vi "Launch Process.vi"(8 "error in (no error)":errorcluster, 10 "TopLevel":refnum<class "TopLevel.lvclass">, 11 "Database in":refnum<class "Database.lvclass">) -> (0 "error out":errorcluster, 1 "timed out?":bool, 2 "sync from process?":bool, 3 "Database out":refnum<class "Database.lvclass">)   [LabVIEW 2022 SP3, in "Database.lvclass"]
doc: "Developed by Kevin Thompson\nkevin@thompsonengineering.net\n\nCopyright 2018\nThompson Engineering, LLC"
uses:
  Database.lvclass
  TopLevel/TopLevel.lvclass
  Process.vi
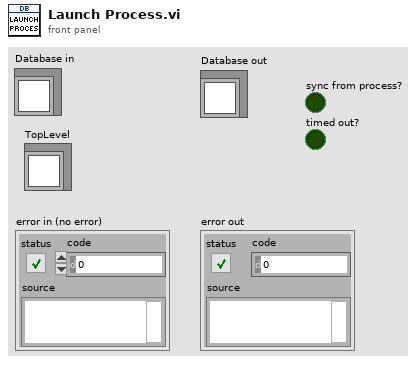
[diagram p1: front panel]
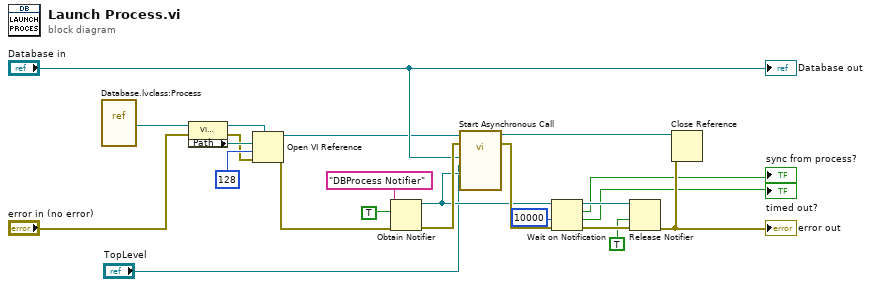
[diagram p0: block diagram]
diagram:
  n1 = vi-ref "Database.lvclass:Process.vi"() -> (w10:refnum<vi>)
  n2 = property class="VI (strict)"(reference=w10, error in="error in (no error)") -> (reference out=w8:refnum<vi>, error out=w17:errorcluster, "Path"=w22:path)
  n3 = Open VI Reference(type specifier VI Refnum (for type only)=w8, vi path=w22, options=128, error in (no error)=w17) -> (vi reference=w7:refnum<vi>, error out=w2:errorcluster)  [unwired: 2 in]
  n4 = Obtain Notifier(name (unnamed)="DBProcess Notifier", notification data type=TRUE, error in (no error)=w2) -> (notifier out=w15:refnum<notifier>, error out=w19:errorcluster)  [unwired: 1 in, 1 out]
  n5 = call-by-ref "Start Asynchronous Call"(reference=w7, error in=w19, "process sync"=w15, "TopLevel"="TopLevel", "Database in"="Database in") -> (reference out=w12:refnum<vi>, error out=w18:errorcluster)  [unwired: 9 in]
  n6 = Wait on Notification(notifier=w15, timeout in ms (-1)=10000, error in (no error)=w18) -> (notifier out=w13:refnum<notifier>, notification=→"sync from process?":bool, timed out?=→"timed out?":bool, error out=w14:errorcluster)  [unwired: 1 in]
  n7 = Release Notifier(notifier=w13, force destroy? (F)=TRUE, error in (no error)=w14) -> (error out=w23:errorcluster)  [unwired: 2 out]
  "error out" <- w23
  n8 = Close Reference(reference=w12, error in (no error)=w23) -> ()  [unwired: 1 out]
  "Database out" <- "Database in"
